vi "_get_selection_type_name.vi"(8 "error in":errorcluster, 11 "vs_tree_control in":refnum<class "vs_tree_control.lvclass">) -> (0 "error out":errorcluster, 2 "TypeName":string, 3 "vs_tree_control out":refnum<class "vs_tree_control.lvclass">)   [LabVIEW 2020, in "vs_tree_control.lvclass"]
uses:
  vs_tree_control.lvclass
  vs_tree_control.lvclass/vs_tree_control.ctl
  NationalInstruments.VeriStand.SystemStorageUI
  NationalInstruments.VeriStand.SystemStorage
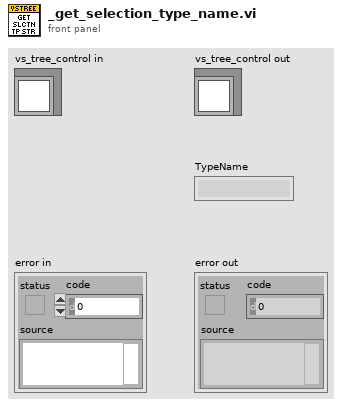
[diagram p1: front panel]
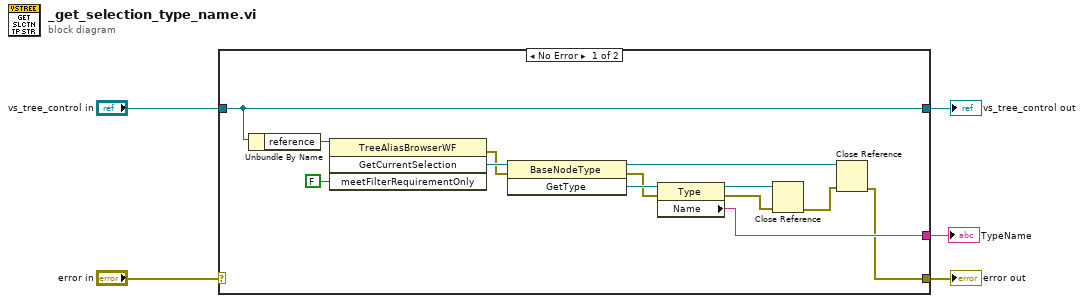
[diagram p0: block diagram]
diagram:
  n1 = case shown="No Error" "error in" {
    selector: "error in" -> [_ w20]
    tunnel: [w6 w20] -> w4
    tunnel: [w15 w19] -> w2
    tunnel: "vs_tree_control in" -> [w15 w19]
    tunnel: [w13 _] -> w1
    frame No Error {
      n2 = Unbundle By Name(w15) -> ("reference"=w14:refnum<k24>)
      n3 = invoke class="TreeAliasBrowserWF" method="GetCurrentSelection"(reference=w14, "meetFilterRequirementOnly"=FALSE) -> (error out=w7:errorcluster, "GetCurrentSelection"=w17:refnum<k24>)  [unwired: 2 in, 2 out]
      n4 = invoke class="BaseNodeType" method="GetType"(reference=w17, error in=w7) -> (reference out=w12:refnum<k24>, error out=w8:errorcluster, "GetType"=w18:refnum<k24>)  [unwired: 1 in]
      n5 = property class="Type"(reference=w18, error in=w8) -> (reference out=w11:refnum<k24>, error out=w9:errorcluster, "Name"=w13:string)
      n6 = Close Reference(reference=w11, error in (no error)=w9) -> (error out=w10:errorcluster)
      n7 = Close Reference(reference=w12, error in (no error)=w10) -> (error out=w6:errorcluster)
    }
    frame Error {
    }
  }
  "error out" <- w4
  "vs_tree_control out" <- w2
  "TypeName" <- w1
